vi "Query Regulation Gain Capabilities.vi"(0 "VISA resource name":refnum<visa-resource-name>, 11 "error in (no error)":errorcluster) -> (4 "VISA resource name out":refnum<visa-resource-name>, 6 "Minimum":dbl, 8 "Nominal":dbl, 10 "Maximum":dbl, 15 "error out":errorcluster)   [LabVIEW 2012, in "NH Research Regenerative Test Series.lvlib"]
doc: "This will query the absolute minimum and maximum legal values for regulation gain and the nominal (default) value."
uses:
  <instrlib>/NH Research Regenerative Test Series/NH Research Regenerative Test Series.lvlib
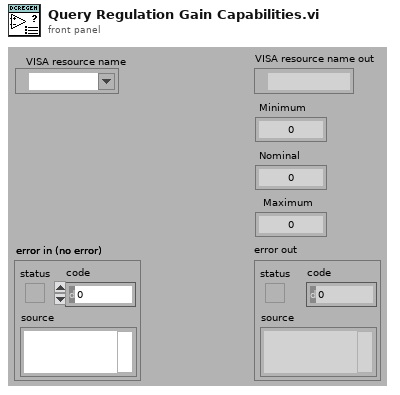
[diagram p1: front panel]
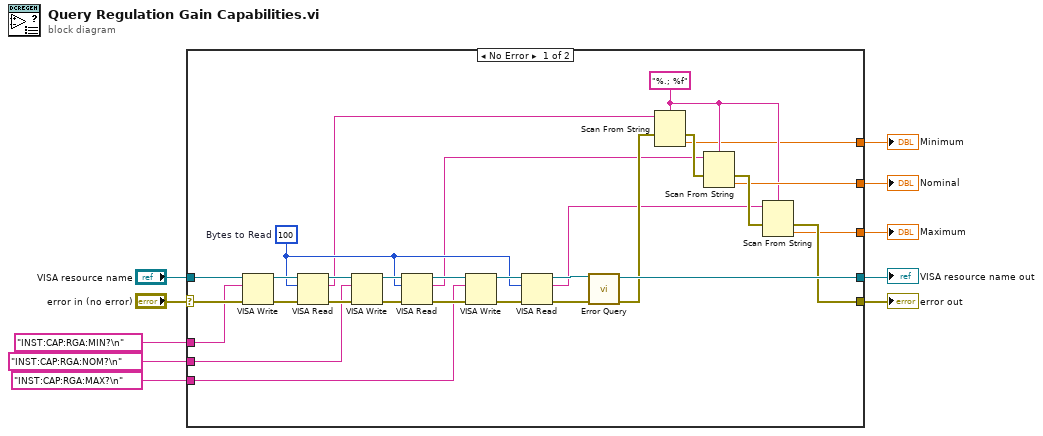
[diagram p0: block diagram]
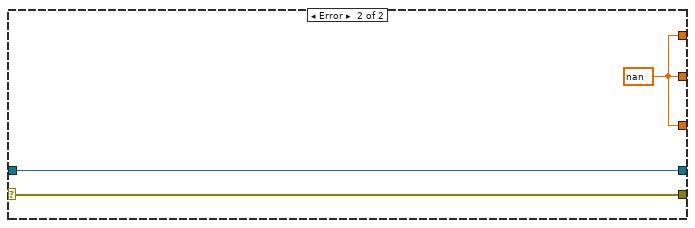
[diagram p2: hidden frame]
diagram:
  n1 = case shown="No Error" "error in (no error)" {
    selector: "error in (no error)" -> [w38 w43]
    tunnel: [w18 w43] -> w9
    tunnel: [w36 w42] -> w7
    tunnel: "VISA resource name" -> [w37 w42]
    tunnel: "INST:CAP:RGA:MIN?\n" ("write buffer") -> [w28 _]
    tunnel: "INST:CAP:RGA:NOM?\n" ("write buffer") -> [w27 _]
    tunnel: "INST:CAP:RGA:MAX?\n" ("write buffer") -> [w26 _]
    tunnel: [w17 w41] -> w2
    tunnel: [w16 w41] -> w1
    tunnel: [w11 w41] -> w3
    frame No Error {
      w12 = "%.; %f" ("format string")
      w23 = u32 100  # Bytes to Read
      n2 = VISA Write(VISA resource name=w37, write buffer=w28, error in (no error)=w38) -> (VISA resource name out=w39:refnum<visa-resource-name>, error out=w40:errorcluster)  [unwired: 1 out]
      n3 = VISA Read(VISA resource name=w39, byte count=w23, error in (no error)=w40) -> (VISA resource name out=w25:refnum<visa-resource-name>, read buffer=w15:string, error out=w30:errorcluster)  [unwired: 1 out]
      n4 = VISA Write(VISA resource name=w25, write buffer=w27, error in (no error)=w30) -> (VISA resource name out=w33:refnum<visa-resource-name>, error out=w34:errorcluster)  [unwired: 1 out]
      n5 = VISA Read(VISA resource name=w33, byte count=w23, error in (no error)=w34) -> (VISA resource name out=w24:refnum<visa-resource-name>, read buffer=w14:string, error out=w29:errorcluster)  [unwired: 1 out]
      n6 = VISA Write(VISA resource name=w24, write buffer=w26, error in (no error)=w29) -> (VISA resource name out=w31:refnum<visa-resource-name>, error out=w32:errorcluster)  [unwired: 1 out]
      n7 = VISA Read(VISA resource name=w31, byte count=w23, error in (no error)=w32) -> (VISA resource name out=w21:refnum<visa-resource-name>, read buffer=w13:string, error out=w22:errorcluster)  [unwired: 1 out]
      n8 = call <instrlib>:"Error Query.vi"("VISA resource name"=w21, "error in (no error)"=w22) -> ("VISA resource name out"=w36:refnum<visa-resource-name>, "error out"=w35:errorcluster)  [unwired: 10 in, 2 out]
      n9 = Scan From String(format string=w12, input string=w15, error in=w35) -> (error out=w20:errorcluster, output 1=w11:dbl)  [unwired: 2 in, 2 out]
      n10 = Scan From String(format string=w12, input string=w14, error in=w20) -> (error out=w19:errorcluster, output 1=w17:dbl)  [unwired: 2 in, 2 out]
      n11 = Scan From String(format string=w12, input string=w13, error in=w19) -> (error out=w18:errorcluster, output 1=w16:dbl)  [unwired: 2 in, 2 out]
    }
    frame Error {
      w41 = nan
    }
  }
  "error out" <- w9
  "VISA resource name out" <- w7
  "Minimum" <- w3
  "Nominal" <- w2
  "Maximum" <- w1
